vi "Edit and Save Key Variable.vi"(8 "error in":errorcluster) -> ()   [LabVIEW 2015]
uses:
  <vilib>/Utility/config.llb/NI_LVConfig.lvlib
  <vilib>/Rock Robotics/Network Tables/NT Write String Array.vi
  <vilib>/Rock Robotics/Network Tables/NT Read Boolean.vi
  <vilib>/Rock Robotics/Network Tables/NT Read String Array.vi
  <vilib>/Utility/config.llb/Write Key (String).vi
panel:
  in  "Preferences":string[][](array[string])
  in  "Cancel":bool
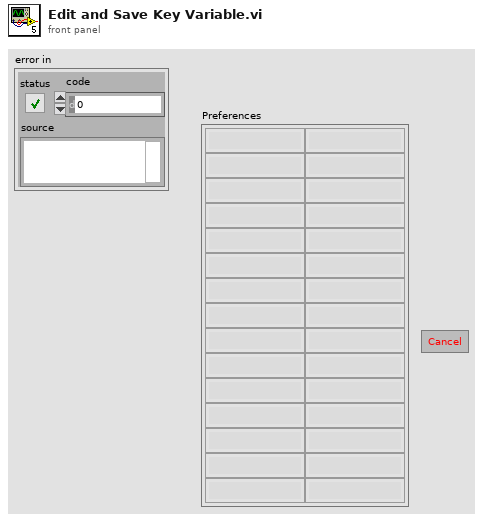
[diagram p1: front panel]
types:
  T1 = typedef "NI_LVConfig.lvlib/Config Data RefNum.ctl" = refnum<k1>
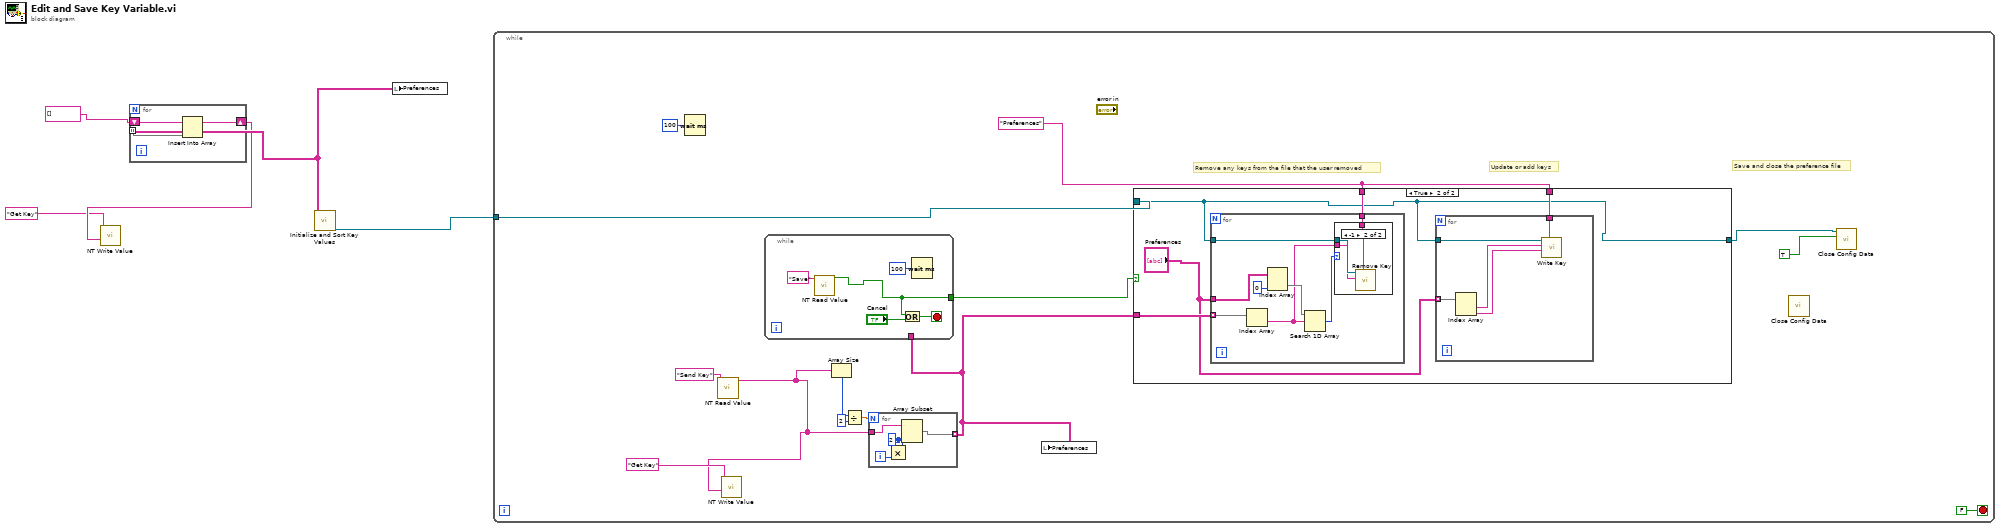
[diagram p0: block diagram]
diagram:
  n1 = call "Initialize and Sort Key Values.vi"() -> ("refnum"=w1:T1, "Preferences"=w5:string[][])  [unwired: 10 in]
  n2 = for {
    tunnel: w5 -> [w7] mode=indexing
    shift-right: [w6] -> w4
    shift-left: string[] [] -> [w8]
    n3 = Insert Into Array(array=w8, new element=w7) -> (w6:string[])  [unwired: 1 in]
  }
  n4 = call-poly <vilib>:"NT Write Value.vi"("String Array"=w4, "Name"="Get Key") -> ()  [unwired: 9 in, 1 out]
  n5 = local write "Preferences"(w5) -> ()
  n6 = while {
    tunnel: w1 -> [w13]
    stop <- FALSE stop-if-true
    w22 = "Preferences" ("section")
    # "Save and close the preference file"
    # "Update or add keys"
    # "Remove any keys from the file that the user removed"
    n7 = Wait (ms)(milliseconds to wait=u32 100) -> ()  [unwired: 1 out]
    n8 = call-poly <vilib>:"NT Read Value.vi"("Name"="Send Key") -> ("String Array"=w15:string[])  [unwired: 9 in, 1 out]
    n9 = call-poly <vilib>:"NT Write Value.vi"("String Array"=w15, "Name"="Get Key") -> ()  [unwired: 9 in, 1 out]
    n10 = Array Size(array=w15) -> (size(s)=w19:i32)
    n11 = Divide(x=w19, y=2) -> (x/y=w20:dbl)
    n12 = for {
      N: w20 -> [_]
      tunnel: w15 -> [w27]
      tunnel: [w26] -> w11 mode=indexing
      i -> [w25]
      w24 = 2 ("length")
      n13 = Multiply(x=w24, y=w25) -> (x*y=w23:i32)
      n14 = Array Subset(array=w27, index=w23, length=w24) -> (w26:string[])
    }
    n15 = while {
      tunnel: [w51] -> w14
      tunnel: w11 -> [_]
      stop <- w53 stop-if-true
      n16 = call-poly <vilib>:"NT Read Value.vi"("Name"="Save") -> ("Boolean"=w51:bool)  [unwired: 9 in, 1 out]
      n17 = Or(x=w51, y="Cancel") -> (x .or. y?=w53:bool)
      n18 = Wait (ms)(milliseconds to wait=u32 100) -> ()  [unwired: 1 out]
    }
    n19 = local write "Preferences"(w11) -> ()
    n20 = case shown="True" w14 {
      tunnel: w13 -> [w28 w29]
      tunnel: w11 -> [_ w33]
      tunnel: w22 -> [_ w32]
      tunnel: [w28 w29] -> w9
      tunnel: w22 -> [_ w31]
      frame False {
      }
      frame True {
        n21 = for {
          tunnel: w29 -> [w43]
          tunnel: w33 -> [w46] mode=indexing
          tunnel: w32 -> [w42]
          tunnel: "Preferences" -> [w39]
          n22 = Index Array(array=w46) -> (element=w41:string)  [unwired: 1 in]
          n23 = Index Array(array=w39, index (col)=0 ("disabled index (col)")) -> (element=w44:string[])  [unwired: 1 in]
          n24 = Search 1D Array(1D array=w44, element=w41) -> (index of element=w40:i32)  [unwired: 1 in]
          n25 = case shown="-1" w40 {
            tunnel: w43 -> [_ w49]
            tunnel: w42 -> [_ w48]
            tunnel: w41 -> [_ w47]
            frame 0, Default {
            }
            frame -1 {
              n26 = call <vilib>:"Remove Key.vi"("section"=w48, "key"=w47, "refnum"=w49) -> ()  [unwired: 6 in, 3 out]
            }
          }
        }
        n27 = for {
          tunnel: "Preferences" -> [w38] mode=indexing
          tunnel: w29 -> [w34]
          tunnel: w31 -> [w37]
          n28 = Index Array(array=w38) -> (element #1=w36:string, element #2=w35:string)  [unwired: 2 in]
          n29 = call-poly <vilib>:"Write Key.vi"("section"=w37, "value"=w35, "key"=w36, "refnum"=w34) -> ()  [unwired: 5 in, 3 out]
        }
      }
    }
    n30 = call <vilib>:"Close Config Data.vi"() -> ()  [unwired: 10 in, 2 out]
    n31 = call <vilib>:"Close Config Data.vi"("write file if changed (T)"=TRUE, "refnum"=w9) -> ()  [unwired: 8 in, 2 out]
  }
